vi "View Specifications.vi"(8 "error in (no error)":errorcluster, 10 "configuration file path":path) -> (0 "error out":errorcluster, 2 "Results Table":string[][](array[string]))   [LabVIEW 2018]
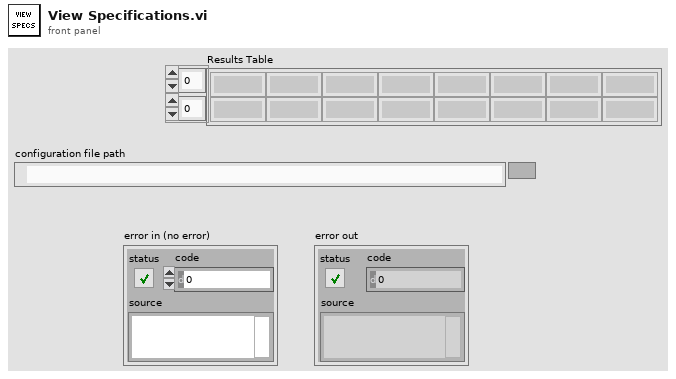
[diagram p1: front panel]
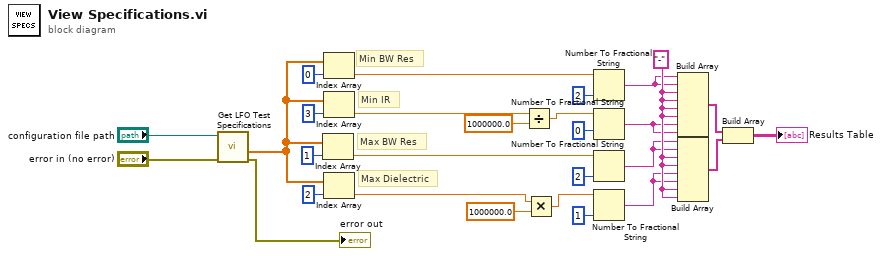
[diagram p0: block diagram]
diagram:
  w28 = "-" ("element")
  # "Min IR"
  # "Max BW Res"
  # "Max Dielectric"
  # "Min BW Res"
  n1 = call "Get LFO Test Specifications.vi"("error in (no error)"="error in (no error)", "configuration file path"="configuration file path") -> ("error out"=→"error out":errorcluster, "Test Specifications"=w20:dbl[])  [unwired: 7 in, 1 out]
  n2 = Index Array(array=w20, index=1) -> (element=w3:dbl)
  n3 = Index Array(array=w20, index=0) -> (element=w19:dbl)
  n4 = Index Array(array=w20, index=3) -> (element=w2:dbl)
  n5 = Index Array(array=w20, index=2) -> (element=w7:dbl)
  n6 = Divide(x=w2, y=1000000.0) -> (x/y=w1:dbl)
  n7 = Multiply(x=w7, y=1000000.0) -> (x*y=w6:dbl)
  n8 = Number To Fractional String(number=w19, precision (6)=i16 2) -> (F-format string=w18:string)  [unwired: 2 in]
  n9 = Number To Fractional String(number=w1, precision (6)=i16 0) -> (F-format string=w15:string)  [unwired: 2 in]
  n10 = Number To Fractional String(number=w3, precision (6)=i16 2) -> (F-format string=w16:string)  [unwired: 2 in]
  n11 = Number To Fractional String(number=w6, precision (6)=i16 1) -> (F-format string=w17:string)  [unwired: 2 in]
  n12 = Build Array(w18, w18, w28, w28, w28, w28, w15, w15) -> (w27:string[])
  n13 = Build Array(w16, w16, w28, w28, w17, w17, w28, w28) -> (w26:string[])
  n14 = Build Array(w27, w26) -> (→"Results Table":string[][])
